vi "User Interface.vi"(8 "error in":errorcluster, 11 "User Interface in":refnum<class "User Interface.lvclass">=refnum) -> (0 "error out":errorcluster, 3 "User Interface out":refnum<class "User Interface.lvclass">)   [LabVIEW 2020, in "RDMA.lvlib" / "RDMA Transfer Rx User Interface.lvclass"]
uses:
  RDMA Transfer Rx User Interface.lvclass
  Configuration/Rx Transfer/RDMA Transfer Rx Configuration.lvclass
  DSF Core.lvlibp/Classes/User Interface/User Interface.lvclass
panel:
  in  "Local Address":string
  in  "Local Port":u16
  # "RDMA Plugin Settings"
  # "* The local address field must be in IP dot notation. \n   Example: 10.0.53.23"
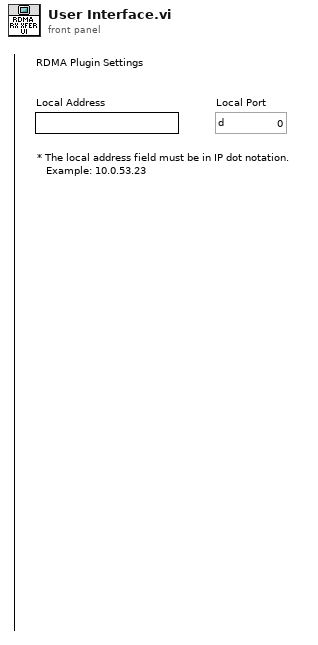
[diagram p1: front panel]
types:
  T1 = typedef "RDMA.lvlib/RDMA Transfer Rx Configuration.lvclass/Rx Transfer Settings.ctl" = cluster{"local address":u32, "local port":u16}
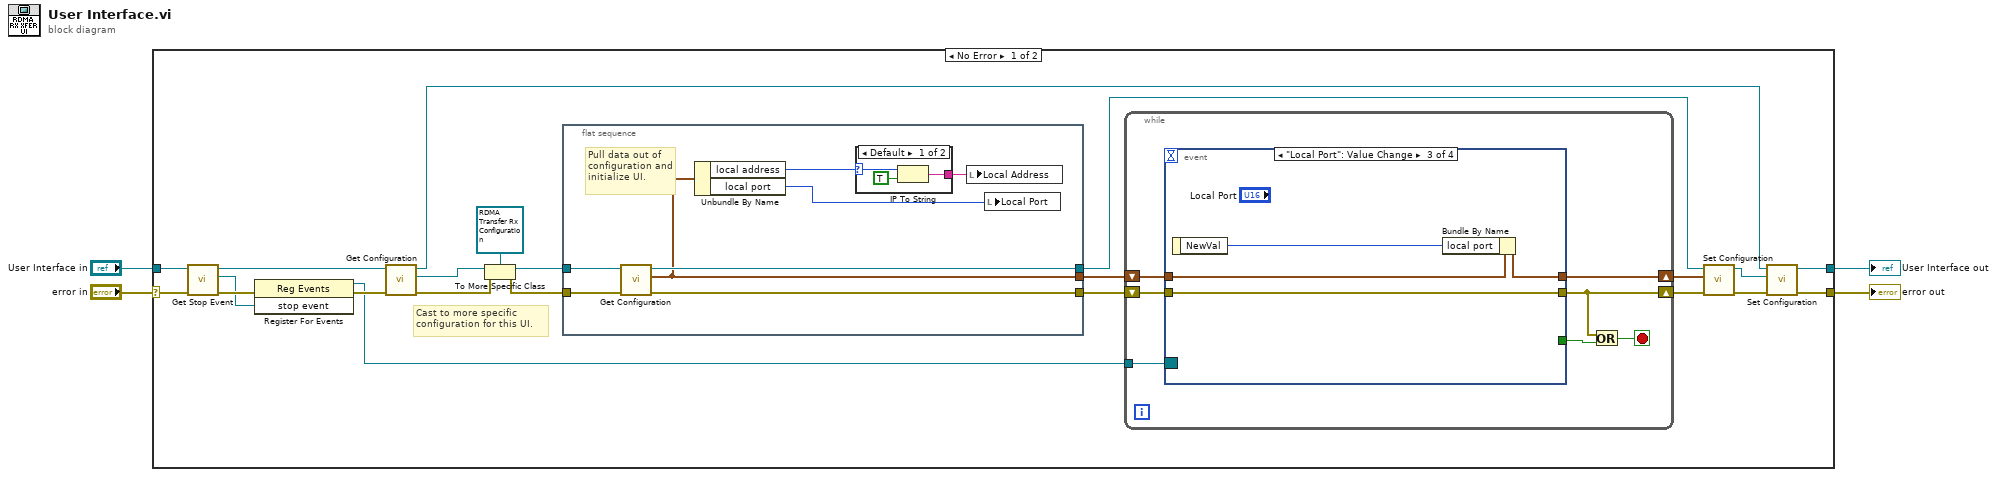
[diagram p0: block diagram]
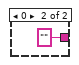
[diagram p2: hidden frame]
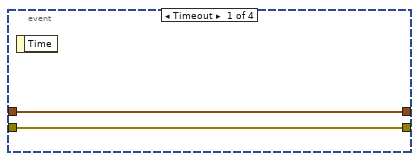
[diagram p3: hidden frame]
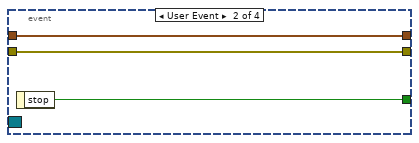
[diagram p4: hidden frame]
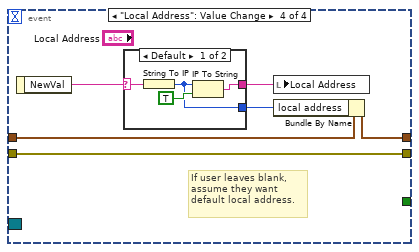
[diagram p5: hidden frame]
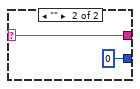
[diagram p6: hidden frame]
diagram:
  n1 = case shown="No Error" "error in" {
    selector: "error in" -> [w23 w68]
    tunnel: [w14 w68] -> w4
    tunnel: "User Interface in" -> [w22 w67]
    tunnel: [w13 w67] -> w1
    frame No Error {
      # "Cast to more specific configuration for this UI."
      n2 = call "Get Stop Event.vi"("error in (no error)"=w23, "User Interface in"=w22) -> ("error out"=w21:errorcluster, "stop event"=w20:refnum<user-event>, "User Interface out"=w19:refnum<class "User Interface.lvclass">)  [unwired: 7 in]
      n3 = register-events(error in=w21, w20) -> (reference out=w17:refnum<event-registration>, error out=w18:errorcluster)  [unwired: 1 in]
      n4 = call "Get Configuration.vi"("error in (no error)"=w18, "User Interface in"=w19) -> ("error out"=w16:errorcluster, "configuration"=w15:refnum<class "Configuration.lvclass">, "User Interface out"=w12:refnum<class "User Interface.lvclass">)  [unwired: 7 in]
      n5 = To More Specific Class(target class=refnum<class "RDMA Transfer Rx Configuration.lvclass"> refnum ("DSF Core.lvlib:UDP Transfer Rx Configuration.lvclass"), reference=w15, error in=w16) -> (specific class reference=w26:refnum<class "RDMA Transfer Rx Configuration.lvclass">, error out=w24:errorcluster)
      n6 = flat-sequence {
        tunnel: [w32] -> w25
        tunnel: w24 -> [w34]
        tunnel: w26 -> [w33]
        tunnel: [w30] -> w6
        tunnel: [w29] -> w10
        frame #0 {
          # "Pull data out of configuration and initialize UI."
          n7 = call "Get Configuration.vi"("error in"=w34, "RDMA Transfer Rx Configuration in"=w33) -> ("error out"=w32:errorcluster, "transfer settings"=w29:T1, "RDMA Transfer Rx Configuration out"=w30:refnum<class "RDMA Transfer Rx Configuration.lvclass">)  [unwired: 7 in]
          n8 = Unbundle By Name(w29) -> ("local address"=w28:u32, "local port"=w27:u16)
          n9 = case shown="Default" w28 {
            selector: w28 -> [w35 _]
            tunnel: [w37 "" ("name")] -> w31
            frame Default {
              n10 = IP To String(1:TRUE ("dot notation? (F)"), 2:w35) -> (0:w37:string)
            }
            frame 0 {
            }
          }
          n11 = local write "Local Address"(w31) -> ()
          n12 = local write "Local Port"(w27) -> ()
        }
      }
      n13 = while {
        tunnel: w17 -> [w45]
        shift-right: [w43] -> w9
        shift-left: w25 -> [w44]
        shift-right: [w39] -> w7
        shift-left: w10 -> [w40]
        stop <- w42 stop-if-true
        n14 = event shown="[2] \"Local Port\": Value Change" {
          selector: w45 -> [_ _ _ _]
          dyn-events: _ -> [_ _ _ _]
          timeout: _ -> [_ _ _ _]
          tunnel: [_ w49 _ _] -> w41
          tunnel: w44 -> [w47 w50 w54 w57]
          tunnel: [w47 w50 w54 w57] -> w43
          tunnel: w40 -> [w46 w48 w53 w58]
          tunnel: [w46 w48 w52 w60] -> w39
          event Timeout {
            n15 = event-data() -> ()  [unwired: 1 in, 1 out]
          }
          event User Event {
            n16 = event-data() -> ("stop"=w49:bool)  [unwired: 1 in]
          }
          event "Local Port": Value Change {
            n17 = event-data() -> ("NewVal"=w51:u16)  [unwired: 1 in]
            n18 = Bundle By Name(cluster=w53, "local port"=w51) -> (w52:T1)
          }
          event "Local Address": Value Change {
            # "If user leaves blank, assume they want default local address."
            n19 = event-data() -> ("NewVal"=w55:string)  [unwired: 1 in]
            n20 = case shown="Default" w55 {
              selector: w55 -> [w61 w65]
              tunnel: [w64 w65] -> w59
              tunnel: [w62 u32 0] -> w56
              frame Default {
                n21 = String To IP(1:w61) -> (0:w62:u32)
                n22 = IP To String(1:TRUE ("dot notation? (F)"), 2:w62) -> (0:w64:string)
              }
              frame "" {
              }
            }
            n23 = local write "Local Address"(w59) -> ()
            n24 = Bundle By Name(cluster=w58, "local address"=w56) -> (w60:T1)
          }
        }
        n25 = Or(x=w43, y=w41) -> (x .or. y?=w42:bool)
      }
      n26 = call "Set Configuration.vi"("error in"=w9, "transfer settings"=w7, "RDMA Transfer Rx Configuration in"=w6) -> ("error out"=w8:errorcluster, "RDMA Transfer Rx Configuration out"=w5:refnum<class "RDMA Transfer Rx Configuration.lvclass">)  [unwired: 7 in]
      n27 = call "Set Configuration.vi"("error in (no error)"=w8, "configuration"=w5, "User Interface in"=w12) -> ("error out"=w14:errorcluster, "User Interface out"=w13:refnum<class "User Interface.lvclass">)  [unwired: 7 in]
    }
    frame Error {
    }
  }
  "error out" <- w4
  "User Interface out" <- w1
